vi "CreateLocationsNode.vi"(7 "DOM Document":refnum<k20>, 8 "Error In":errorcluster, 11 "Memory":string[](array[string])) -> (0 "Error Out":errorcluster, 3 "Locations Node":refnum<k20>)   [LabVIEW 2012]
uses:
  libs/LV-Utilities/LV-Utilities.lvlib
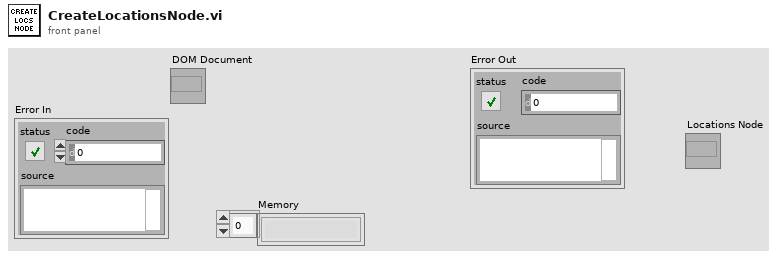
[diagram p1: front panel]
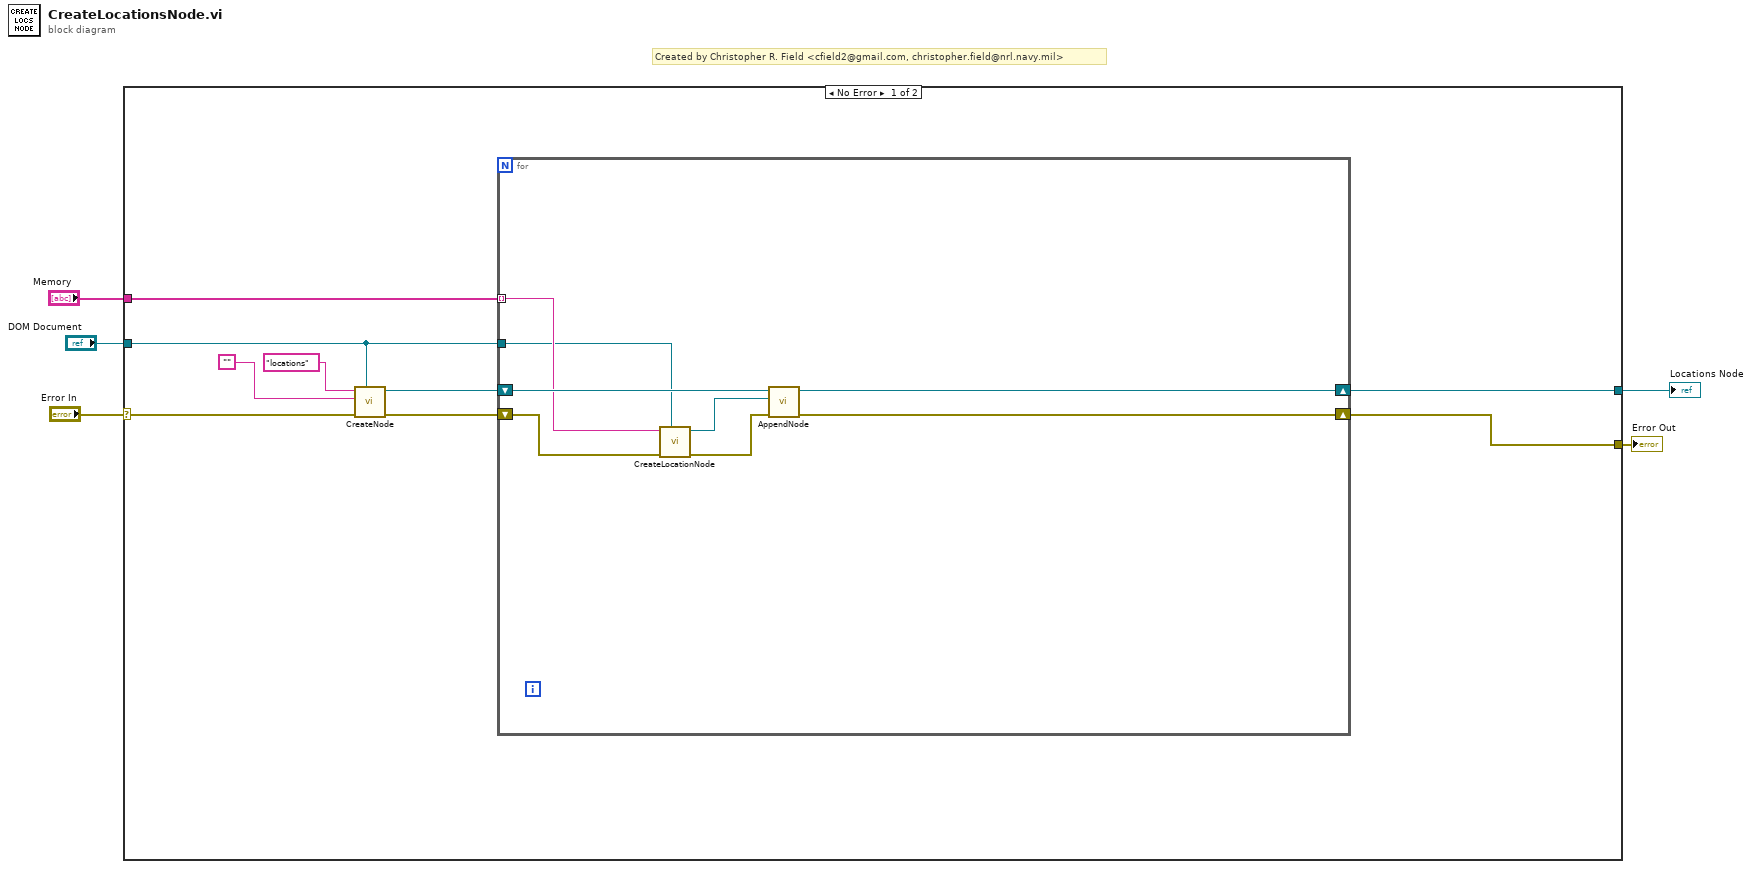
[diagram p0: block diagram]
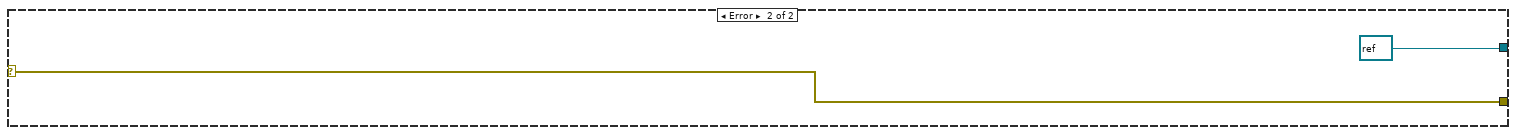
[diagram p2: hidden frame]
diagram:
  # "Created by Christopher R. Field <cfield2@gmail.com, christopher.field@nrl.navy.mil>"
  n1 = case shown="No Error" "Error In" {
    selector: "Error In" -> [w13 w24]
    tunnel: "Memory" -> [w14 _]
    tunnel: "DOM Document" -> [w8 _]
    tunnel: [w7 refnum<k20> refnum ("Channel Node 2")] -> w2
    tunnel: [w6 w24] -> w3
    frame No Error {
      n2 = call "CreateNode.vi"("DOM Document"=w8, "Error In"=w13, "Text"="", "Tag Name"="locations") -> ("Error out"=w12:errorcluster, "Node"=w9:refnum<k20>)  [unwired: 6 in]
      n3 = for {
        tunnel: w14 -> [w19] mode=indexing
        shift-right: [w20] -> w6
        shift-left: w12 -> [w18]
        shift-right: [w21] -> w7
        shift-left: w9 -> [w22]
        tunnel: w8 -> [w15]
        n4 = call "CreateLocationNode.vi"("DOM Document"=w15, "Error In"=w18, "Pattern"=w19) -> ("Error Out"=w17:errorcluster, "Location Node"=w16:refnum<k20>)  [unwired: 7 in]
        n5 = call "AppendNode.vi"("Error In"=w17, "Child Node"=w16, "Parent Node In"=w22) -> ("Error Out"=w20:errorcluster, "Parent Node Out"=w21:refnum<k20>)  [unwired: 7 in]
      }
    }
    frame Error {
    }
  }
  "Error Out" <- w3
  "Locations Node" <- w2
